vi "satuModule.vi"(1 "min":dbl, 2 "input":dbl, 3 "max":dbl) -> (0 "output":dbl)   [LabVIEW 2018]
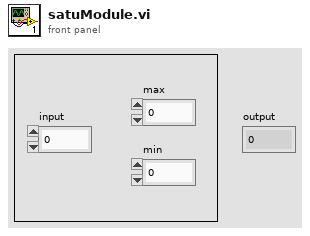
[diagram p1: front panel]
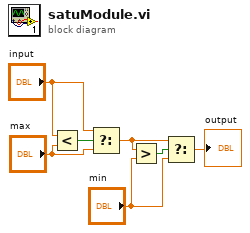
[diagram p0: block diagram]
diagram:
  n1 = Less?(x="input", y="max") -> (x < y?=w7:bool)
  n2 = Select(t="input", s=w7, f="max") -> (s? t:f=w3:dbl)
  n3 = Greater?(x=w3, y="min") -> (0:w4:bool)
  n4 = Select(t=w3, s=w4, f="min") -> (s? t:f=→"output":dbl)
